vi "RSZVB Configure Trigger Settings.vi"(7 "Trigger Delay (0.0 s)":dbl format="%^.3e", 8 "error in (no error)":errorcluster {"code" format="%.0x"}, 9 "Trigger Meas Sequence (0: Sweep)":i32(ring) items=["Sweep", "Sweep Segment", "Point", "Partial Measurement"], 10 "Channel (1)":i32=1, 11 "VISA session":refnum<visa-resource-name>) -> (0 "error out":errorcluster {"code" format="%.0x"}, 3 "dup VISA session":refnum<visa-resource-name>)   [LabVIEW 2011]
doc: "This VI configures the trigger settings.\n\nRemote-control command(s):\nTRIGger<Ch>[:SEQuence]:LINK 'POINT' | 'SWEEP' | 'PPOINT' | 'SEGMENT'\nTRIGger<Ch>[:SEQuence]:HOLDoff"
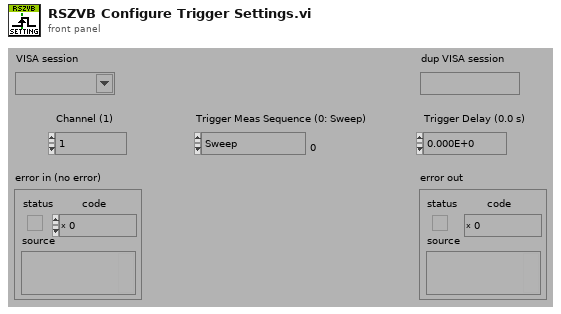
[diagram p1: front panel]
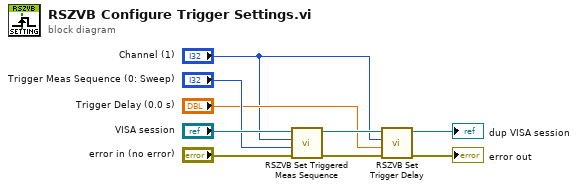
[diagram p0: block diagram]
diagram:
  n1 = call "RSZVB Set Triggered Meas Sequence.vi"("error in (no error)"="error in (no error)", "Trigger Meas Sequence (0: Sweep)"="Trigger Meas Sequence (0: Sweep)", "Channel (1)"="Channel (1)", "VISA session"="VISA session") -> ("error out"=w7:errorcluster, "dup VISA session"=w6:refnum<visa-resource-name>)  [unwired: 6 in]
  n2 = call "RSZVB Set Trigger Delay.vi"("error in (no error)"=w7, "Trigger Delay (0.0 s)"="Trigger Delay (0.0 s)", "Channel (1)"="Channel (1)", "VISA session"=w6) -> ("error out"=→"error out":errorcluster, "dup VISA session"=→"dup VISA session":refnum<visa-resource-name>)  [unwired: 6 in]
